vi "Swap.vi"(8 "error in (no error)":errorcluster, 10 "Other Parameter to Hardware Map in":refnum<class "Parameter to Hardware Map.lvclass">, 11 "Parameter to Hardware Map in":refnum<class "Parameter to Hardware Map.lvclass">) -> (0 "error out":errorcluster, 2 "Other Parameter to Hardware Map out":refnum<class "Parameter to Hardware Map.lvclass">, 3 "Parameter to Hardware Map out":refnum<class "Parameter to Hardware Map.lvclass">)   [LabVIEW 2020, in "RxnRover.lvlib" / "Parameter to Hardware Map.lvclass"]
doc: "Swaps the elements of one Parameter to Hardware Map with another."
uses:
  Parameter to Hardware Map.lvclass
  Parameter to Hardware Map.lvclass/Parameter to Hardware Map.ctl
  Controller/Generic Plugin.lvclass
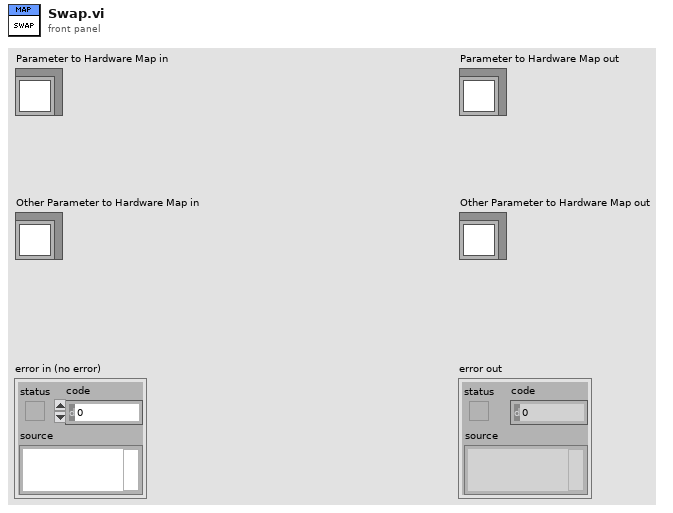
[diagram p1: front panel]
types:
  T1 = typedef "RxnRover.lvlib/Parameter to Hardware Map.lvclass/Pair.ctl" = cluster{"key":string, "values":refnum<class "Generic Plugin.lvclass">[]}
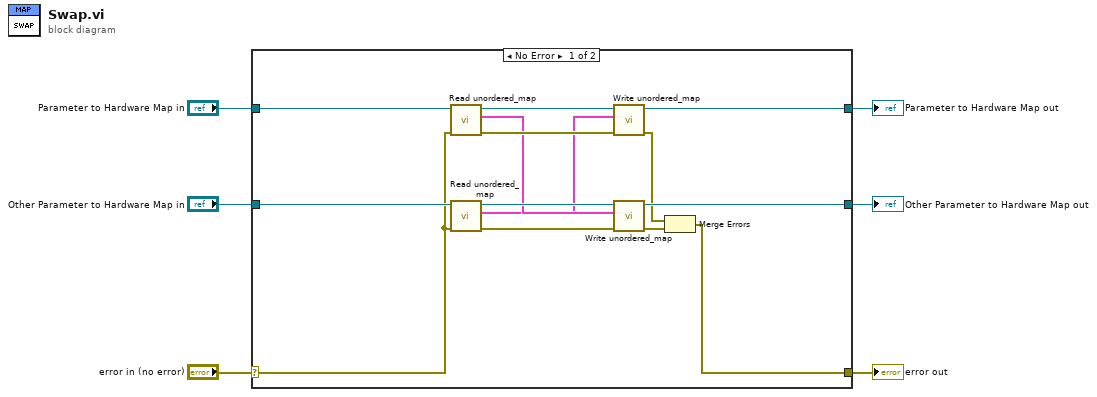
[diagram p0: block diagram]
diagram:
  n1 = case shown="No Error" "error in (no error)" {
    selector: "error in (no error)" -> [w16 w23]
    tunnel: [w8 w23] -> w5
    tunnel: [w15 w22] -> w3
    tunnel: "Parameter to Hardware Map in" -> [w20 w22]
    tunnel: "Other Parameter to Hardware Map in" -> [w19 w21]
    tunnel: [w14 w21] -> w1
    frame No Error {
      n2 = call "Read unordered_map.vi"("error in (no error)"=w16, "Parameter to Hardware Map in"=w20) -> ("error out"=w13:errorcluster, "unordered_map"=w11:T1[], "Parameter to Hardware Map out"=w17:refnum<class "Parameter to Hardware Map.lvclass">)  [unwired: 7 in]
      n3 = call "Read unordered_map.vi"("error in (no error)"=w16, "Parameter to Hardware Map in"=w19) -> ("error out"=w12:errorcluster, "unordered_map"=w10:T1[], "Parameter to Hardware Map out"=w18:refnum<class "Parameter to Hardware Map.lvclass">)  [unwired: 7 in]
      n4 = call "Write unordered_map.vi"("error in (no error)"=w13, "unordered_map"=w10, "Parameter to Hardware Map in"=w17) -> ("error out"=w7:errorcluster, "Parameter to Hardware Map out"=w15:refnum<class "Parameter to Hardware Map.lvclass">)  [unwired: 7 in]
      n5 = call "Write unordered_map.vi"("error in (no error)"=w12, "unordered_map"=w11, "Parameter to Hardware Map in"=w18) -> ("error out"=w9:errorcluster, "Parameter to Hardware Map out"=w14:refnum<class "Parameter to Hardware Map.lvclass">)  [unwired: 7 in]
      n6 = Merge Errors(w7, w9) -> (w8:errorcluster)
    }
    frame Error {
    }
  }
  "error out" <- w5
  "Parameter to Hardware Map out" <- w3
  "Other Parameter to Hardware Map out" <- w1
